vi "Initialize.vi"(4 "stop bits (1.0)":u16(ring)=10 items=["1.0"=10, "1.5"=15, "2.0"=20], 5 "timeout, ms (300)":u32=300, 6 "parity (none)":enum16{"None", "Odd", "Even"}(ring), 7 "address (1)":u8=1, 8 "error in (no error)":errorcluster, 9 "data bits (8)":u16(ring)=8 items=["7"=7, "8"=8], 10 "baud rate (115200)":u32=115200, 11 "port":refnum<visa-resource-name>) -> (0 "error out":errorcluster, 3 "MKS MF1 out":refnum<class "PL MKS MF1 USB.lvclass">)   [LabVIEW 2015, in "PL MKS MF1 USB.lvclass"]
doc: "Initializes connection to device using specified settings."
uses:
  PL MKS MF1 USB.lvclass
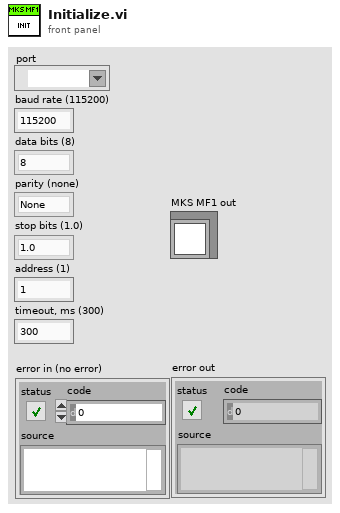
[diagram p1: front panel]
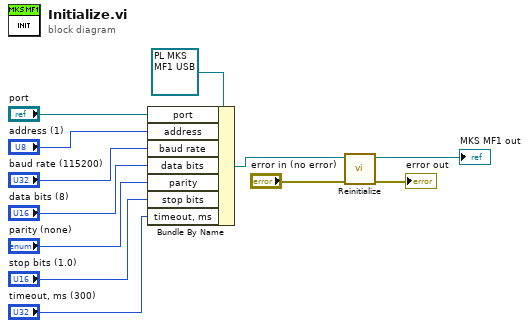
[diagram p0: block diagram]
diagram:
  n1 = Bundle By Name(cluster=refnum<class "PL MKS MF1 USB.lvclass"> refnum, "port"="port", "address"="address (1)", "baud rate"="baud rate (115200)", "data bits"="data bits (8)", "parity"="parity (none)", "stop bits"="stop bits (1.0)", "timeout, ms"="timeout, ms (300)") -> (w12:refnum<class "PL MKS MF1 USB.lvclass">)
  n2 = call "Reinitialize.vi"("error in (no error)"="error in (no error)", "MKS MF1 in"=w12) -> ("error out"=→"error out":errorcluster, "MKS MF1 out"=→"MKS MF1 out":refnum<class "PL MKS MF1 USB.lvclass">)  [unwired: 8 in]
